vi "Configure Device.vi"(8 "error in (no error)":errorcluster, 10 "Max beams":dbl, 11 "Toggle 8 (niDig) in":refnum<class "Toggle 8 (niDig).lvclass">) -> (0 "error out":errorcluster, 3 "Toggle 8 (niDig) out":refnum<class "Toggle 8 (niDig).lvclass">)   [LabVIEW 2020, in "Toggle 8 (niDig).lvclass"]
uses:
  Toggle 8 (niDig).lvclass
panel:
  in  "System Cancel Button":bool
  in  "System OK Button":bool
  out "Meas Write registers":T1(array[cluster]) {"Write Data Array" format="%.0x"}
  out "Init Write registers":T1(array[cluster]) {"Write Data Array" format="%.0x"}
  in  "Measure (extended)":string="0701020100,\n0701020200,\n0701020400,\n0701020800,\n0701021000,\n0701022000,\n0701024000,\n0701020001,\n0701020002,\n0701020004,\n0701020008,\n0701020010,\n0701020020,\n0701020040"
  in  "Init (normal)":string="074000,\n074101,\n07427F,\n07437F,\n074B01,\n074C20,\n074080,\nd200,\n074C31,\nd200"
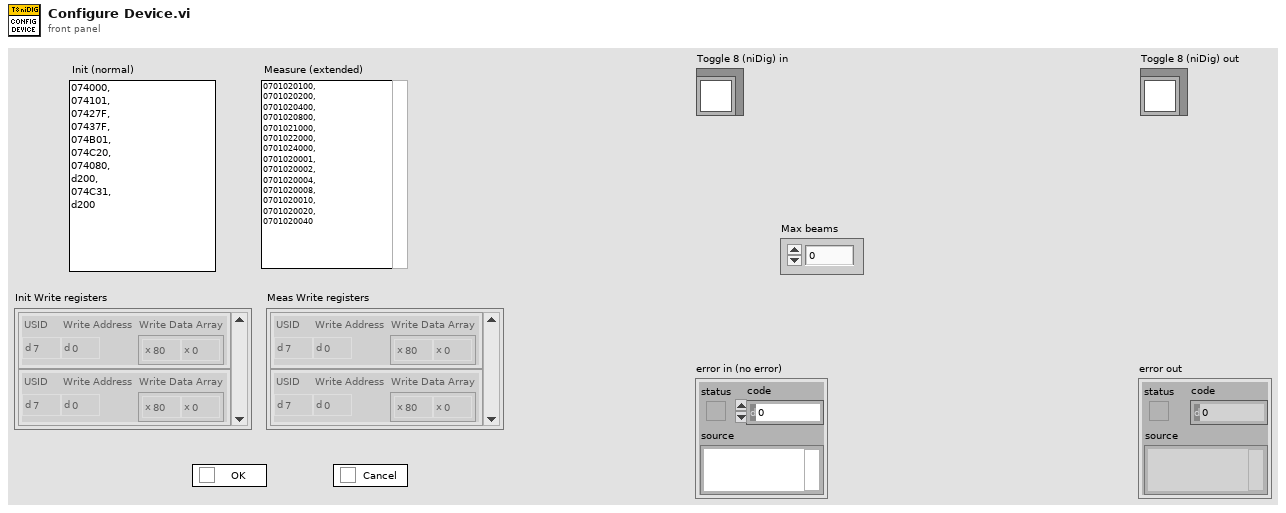
[diagram p1: front panel]
types:
  T1 = cluster{"USID":u8, "Write Address":u8, "Write Data Array":u8[]}[]
  T2 = enum32{"Invalid", "Standard", "Closed", "Hidden", "Minimized", "Maximized"}
  T3 = cluster{"USID":u8, "Write Address":u8, "Write Data Array":u8[]}
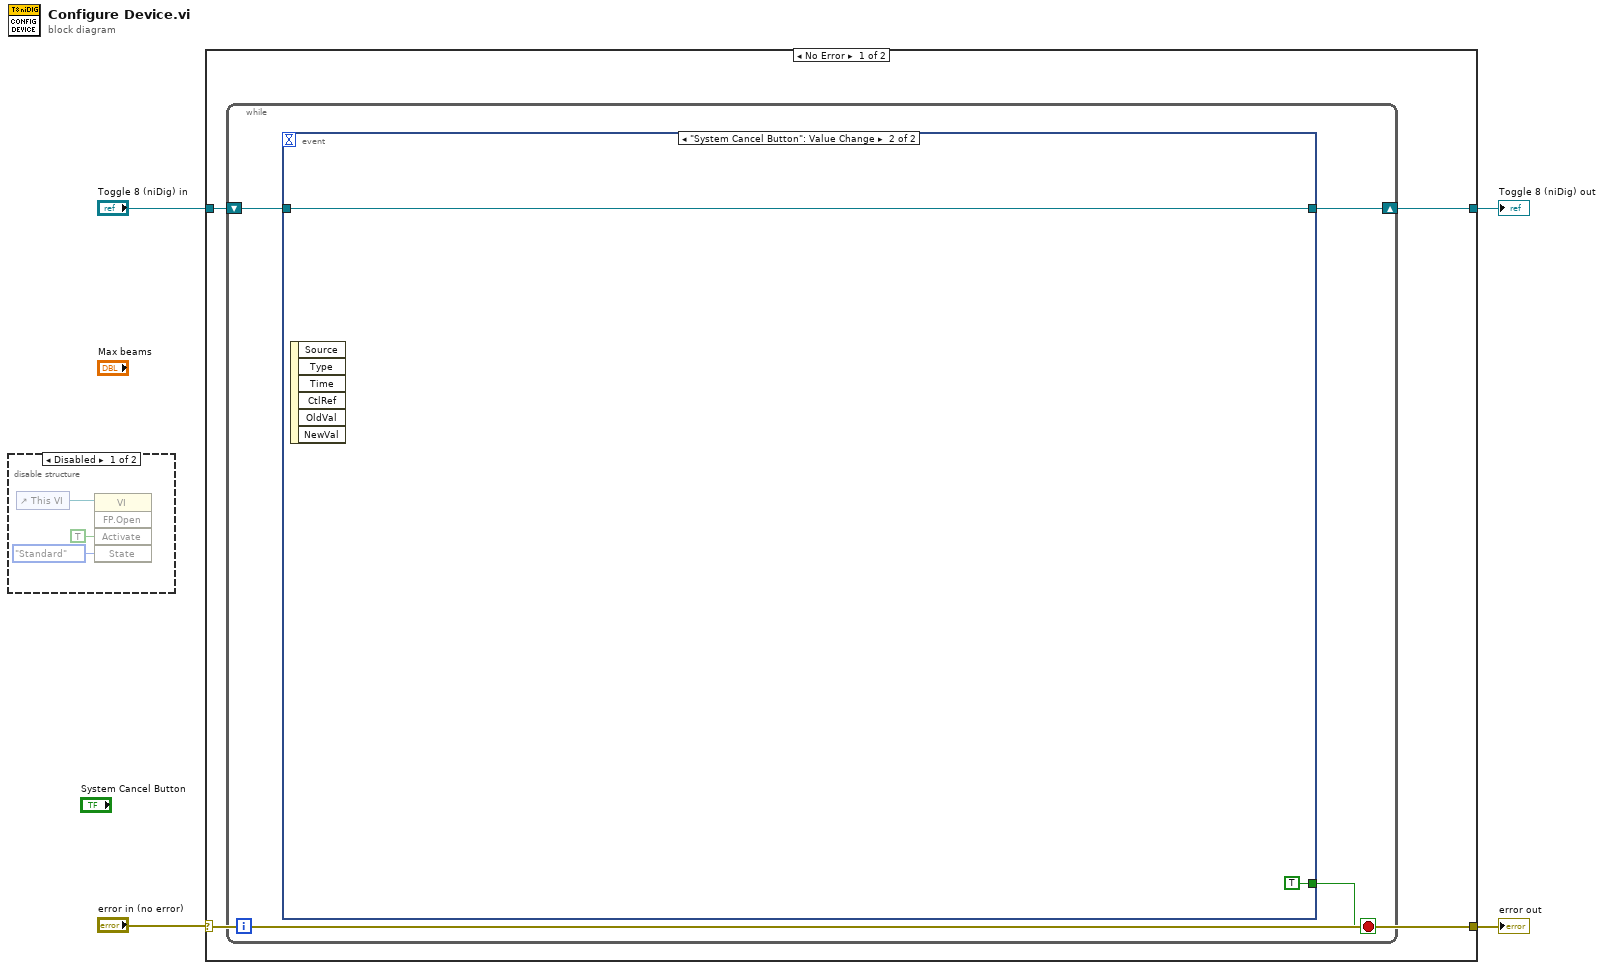
[diagram p0: block diagram]
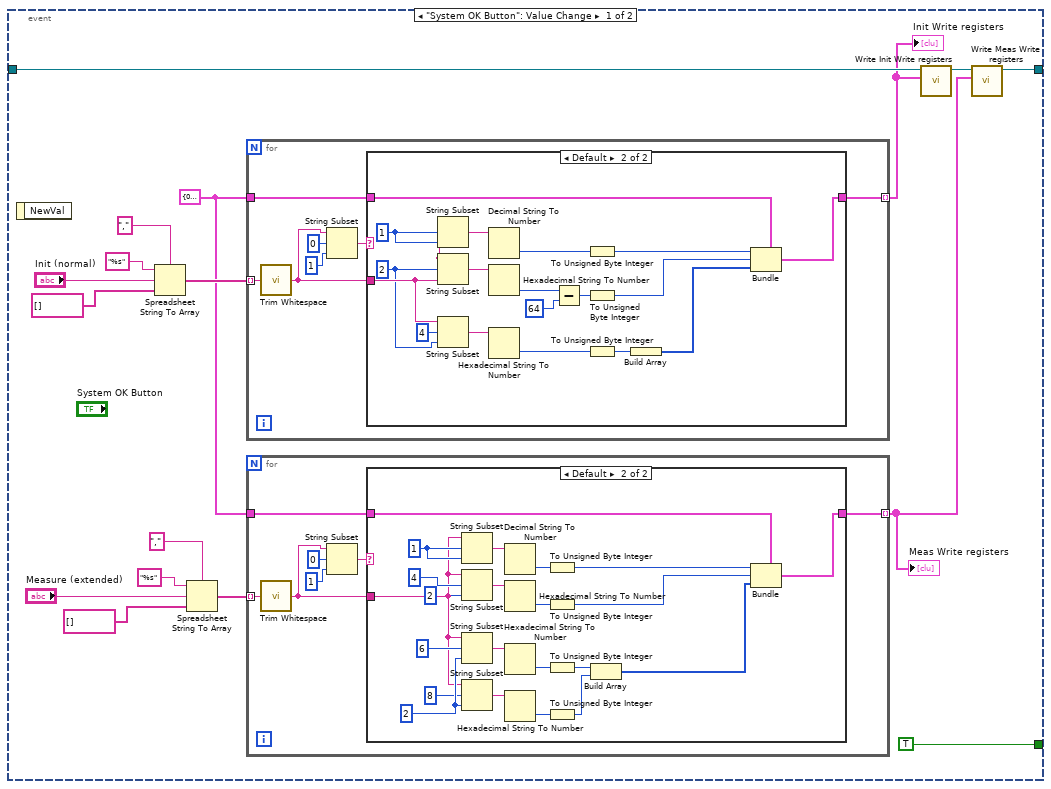
[diagram p3: hidden frame]
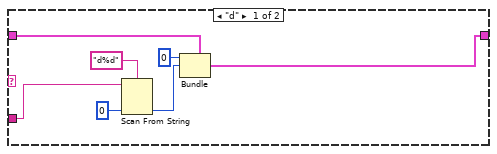
[diagram p4: hidden frame]
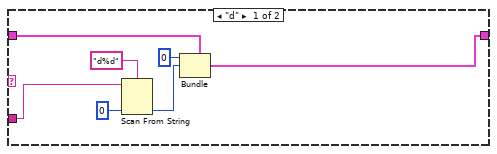
[diagram p5: hidden frame]
diagram:
  n1 = disable-structure shown="Disabled" {
    frame Disabled {
      n2 = control-ref of="This VI"() -> (w7:refnum<vi>)
      n3 = invoke class="VI" method="FP.Open"(reference=w7, "Activate"=TRUE ("Activate?"), "State"=T2."Standard") -> ()  [unwired: 2 in, 5 out]
    }
    frame Enabled {
    }
  }
  n4 = case shown="No Error" "error in (no error)" {
    selector: "error in (no error)" -> [w10 w102]
    tunnel: [w8 w101] -> w4
    tunnel: "Toggle 8 (niDig) in" -> [w9 w101]
    tunnel: [w10 w102] -> w1
    frame No Error {
      n5 = while {
        shift-right: [w12] -> w8
        shift-left: w9 -> [w11]
        stop <- w13 stop-if-true
        n6 = event shown="[1] \"System Cancel Button\": Value Change" {
          selector: _ -> [_ _]
          dyn-events: _ -> [_ _]
          timeout: _ -> [_ _]
          tunnel: [TRUE TRUE] -> w13
          tunnel: [w17 w100] -> w12
          tunnel: w11 -> [w16 w100]
          event "System OK Button": Value Change {
            w25 = T3 {"USID"=0, "Write Address"=0, "Write Data Array"=[]} ("Write register")
            n7 = event-data() -> ()  [unwired: 1 in, 1 out]
            n8 = Spreadsheet String To Array(delimiter (Tab)=",", format string="%s", spreadsheet string="Init (normal)", array type (2D Dbl)=string[] []) -> (array=w28:string[])
            n9 = Spreadsheet String To Array(delimiter (Tab)=",", format string="%s", spreadsheet string="Measure (extended)", array type (2D Dbl)=string[] []) -> (array=w21:string[])
            n10 = for {
              tunnel: w28 -> [w68] mode=indexing
              tunnel: w25 -> [w73]
              tunnel: [w72] -> w15 mode=indexing
              n11 = call <vilib>:"Trim Whitespace.vi"("string"=w68) -> ("trimmed string"=w67:string)  [unwired: 1 in]
              n12 = String Subset(string=w67, offset (0)=0, length (rest)=1 ("length (rest)")) -> (substring=w71:string)
              n13 = case shown="Default" w71 {
                tunnel: w73 -> [w77 w98]
                tunnel: [w76 w93] -> w72
                tunnel: w67 -> [w78 w91]
                frame "d" {
                  n14 = Scan From String(format string="d%d", input string=w78, default 1=u8 0 ("milliseconds to wait")) -> (output 1=w74:u8)  [unwired: 2 in, 3 out]
                  n15 = Bundle(cluster=w77, "USID"=u8 0, "Write Address"=w74) -> (w76:T3)  [unwired: 1 in]
                }
                frame Default {
                  w89 = 2 ("offset (0)")
                  w96 = 1 ("offset (0)")
                  n16 = String Subset(string=w91, offset (0)=w96, length (rest)=w96) -> (substring=w97:string)
                  n17 = String Subset(string=w91, offset (0)=w89, length (rest)=w89) -> (substring=w92:string)
                  n18 = String Subset(string=w91, offset (0)=4, length (rest)=w89) -> (substring=w88:string)
                  n19 = Decimal String To Number(string=w97) -> (number=w86:i32)  [unwired: 2 in, 1 out]
                  n20 = Hexadecimal String To Number(string=w92) -> (number=w95:u32)  [unwired: 2 in, 1 out]
                  n21 = Hexadecimal String To Number(string=w88) -> (number=w82:u32)  [unwired: 2 in, 1 out]
                  n22 = Subtract(x=w95, y=u32 64) -> (x-y=w84:u32)
                  n23 = To Unsigned Byte Integer(number=w86) -> (unsigned 8bit integer=w85:u8)
                  n24 = To Unsigned Byte Integer(number=w84) -> (unsigned 8bit integer=w83:u8)
                  n25 = To Unsigned Byte Integer(number=w82) -> (unsigned 8bit integer=w81:u8)
                  n26 = Build Array(w81) -> (w87:u8[])
                  n27 = Bundle(cluster=w98, "USID"=w85, "Write Address"=w83, "Write Data Array"=w87) -> (w93:T3)
                }
              }
            }
            "Init Write registers" <- w15
            n28 = for {
              tunnel: w21 -> [w32] mode=indexing
              tunnel: w25 -> [w37]
              tunnel: [w36] -> w14 mode=indexing
              n29 = call <vilib>:"Trim Whitespace.vi"("string"=w32) -> ("trimmed string"=w31:string)  [unwired: 1 in]
              n30 = String Subset(string=w31, offset (0)=0, length (rest)=1 ("length (rest)")) -> (substring=w35:string)
              n31 = case shown="Default" w35 {
                tunnel: w37 -> [w41 w66]
                tunnel: [w40 w62] -> w36
                tunnel: w31 -> [w42 w46]
                frame "d" {
                  n32 = Scan From String(format string="d%d", input string=w42, default 1=u8 0 ("milliseconds to wait")) -> (output 1=w38:u8)  [unwired: 2 in, 3 out]
                  n33 = Bundle(cluster=w41, "USID"=u8 0, "Write Address"=w38) -> (w40:T3)  [unwired: 1 in]
                }
                frame Default {
                  w51 = 2 ("length (rest)")
                  w64 = 1 ("offset (0)")
                  n34 = String Subset(string=w46, offset (0)=w64, length (rest)=w64) -> (substring=w65:string)
                  n35 = String Subset(string=w46, offset (0)=4, length (rest)=2 ("length (rest)")) -> (substring=w61:string)
                  n36 = String Subset(string=w46, offset (0)=6, length (rest)=w51) -> (substring=w58:string)
                  n37 = String Subset(string=w46, offset (0)=8, length (rest)=w51) -> (substring=w49:string)
                  n38 = Decimal String To Number(string=w65) -> (number=w56:i32)  [unwired: 2 in, 1 out]
                  n39 = Hexadecimal String To Number(string=w61) -> (number=w63:u32)  [unwired: 2 in, 1 out]
                  n40 = Hexadecimal String To Number(string=w58) -> (number=w53:u32)  [unwired: 2 in, 1 out]
                  n41 = Hexadecimal String To Number(string=w49) -> (number=w48:u32)  [unwired: 2 in, 1 out]
                  n42 = To Unsigned Byte Integer(number=w56) -> (unsigned 8bit integer=w55:u8)
                  n43 = To Unsigned Byte Integer(number=w63) -> (unsigned 8bit integer=w54:u8)
                  n44 = To Unsigned Byte Integer(number=w53) -> (unsigned 8bit integer=w52:u8)
                  n45 = To Unsigned Byte Integer(number=w48) -> (unsigned 8bit integer=w47:u8)
                  n46 = Build Array(w52, w47) -> (w57:u8[])
                  n47 = Bundle(cluster=w66, "USID"=w55, "Write Address"=w54, "Write Data Array"=w57) -> (w62:T3)
                }
              }
            }
            "Meas Write registers" <- w14
            n48 = call-dynamic "Write Init Write registers.vi"("Init Write registers"=w15, "Toggle 8 (niDig) in"=w16) -> ("Toggle 8 (niDig) out"=w18:refnum<class "Toggle 8 (niDig).lvclass">)  [unwired: 9 in]
            n49 = call-dynamic "Write Meas Write registers.vi"("Meas Write registers"=w14, "Toggle 8 (niDig) in"=w18) -> ("Toggle 8 (niDig) out"=w17:refnum<class "Toggle 8 (niDig).lvclass">)  [unwired: 9 in]
          }
          event "System Cancel Button": Value Change {
            n50 = event-data() -> ()  [unwired: 1 in, 6 out]
          }
        }
      }
    }
    frame Error {
    }
  }
  "error out" <- w1
  "Toggle 8 (niDig) out" <- w4
